vi "GPi neuron.vi"(0 "In":bool, 1 "In 2":bool, 2 "In 3":bool, 3 "In 4":bool, 4 "In 5":bool, 5 "In 6":bool, 6 "In 7":bool, 7 "In 8":bool, 9 "In 9":bool, 11 "In 10":bool, 13 "In 11":bool, 15 "In 12":bool, 17 "In 13":bool, 19 "In 14":bool) -> (20 "Out":bool)   [LabVIEW 2014]
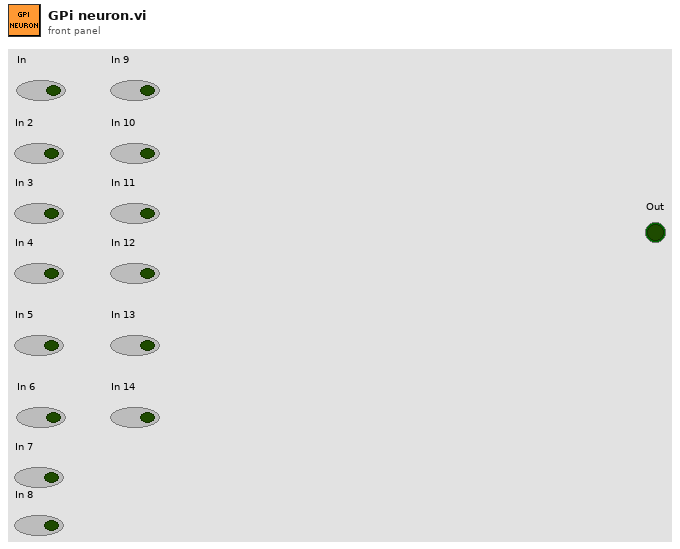
[diagram p1: front panel]
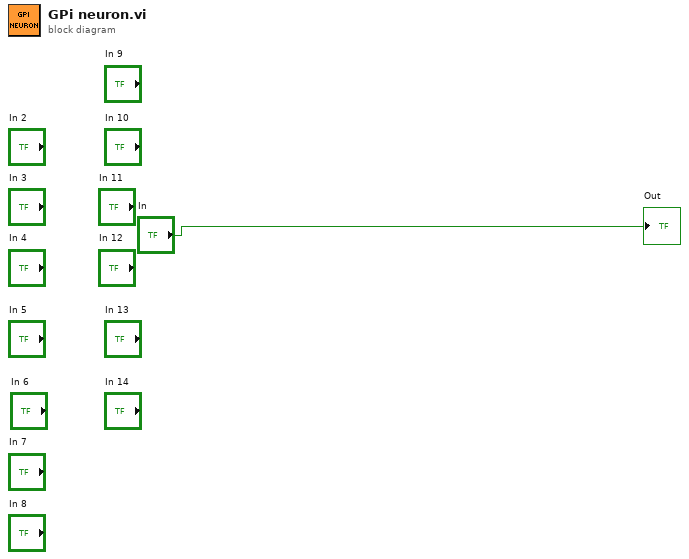
[diagram p0: block diagram]
diagram:
  "Out" <- "In"
